vi "_random_integer.vi"(10 "max":dbl, 11 "min":dbl) -> (3 "output":dbl)   [LabVIEW 2024]
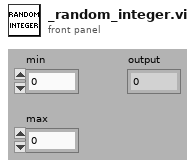
[diagram p1: front panel]
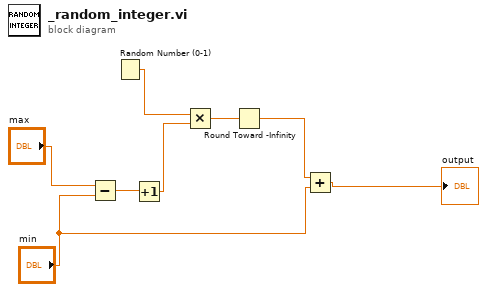
[diagram p0: block diagram]
diagram:
  n1 = Subtract(x="max", y="min") -> (x-y=w7:dbl)
  n2 = Random Number (0-1)() -> (number: 0 to 1=w6:dbl)
  n3 = Increment(x=w7) -> (x+1=w5:dbl)
  n4 = Multiply(x=w6, y=w5) -> (x*y=w4:dbl)
  n5 = Round Toward -Infinity(1:w4) -> (0:w3:dbl)
  n6 = Add(x=w3, y="min") -> (x+y=→"output":dbl)
